vi "postSubDataUE.vi"(6 "newValue (T)":bool=TRUE, 8 "error in (no error)":errorcluster, 9 "value":variant, 10 "subDataSV":T1=enum."captureSpectImage", 11 "Model in":refnum<class "Model.lvclass">) -> (0 "error out":errorcluster, 3 "Model out":refnum<class "Model.lvclass">)   [LabVIEW 2016, in "Model.lvclass"]
uses:
  Model.lvclass
  Typedefs/SubDataSignal.ctl
  Model.lvclass/Model.ctl
  PubSubDataEvent/PubSubDataEvent.lvclass
  Typedefs/SEDSpectrometerTypedefs.lvlib
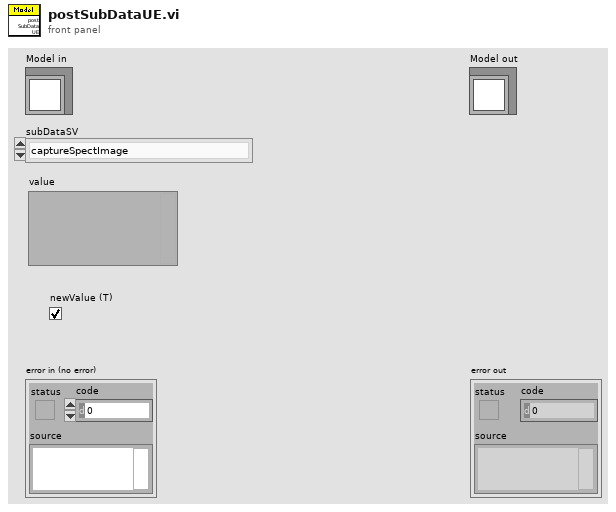
[diagram p1: front panel]
types:
  T1 = typedef "SEDSpectrometerTypedefs.lvlib/SubDataSignal.ctl" = enum16{"disable", "enable", "exit", "standby", "HeartbeatIn", "start", "captureSpectImage"}
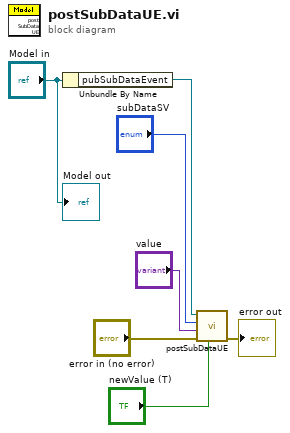
[diagram p0: block diagram]
diagram:
  n1 = Unbundle By Name("Model in") -> ("pubSubDataEvent"=w7:refnum<class "PubSubDataEvent.lvclass">)
  n2 = call "postSubDataUE.vi"("newValue (T)"="newValue (T)", "error in (no error)"="error in (no error)", "value"="value", "subDataSV"="subDataSV", "PubSubDataEvent in"=w7) -> ("error out"=→"error out":errorcluster)  [unwired: 5 in, 1 out]
  "Model out" <- "Model in"
